vi "Read Power DVR FIFO.vi"(8 "error in (no error)":errorcluster, 9 "Timeout (ms)":i32=100, 10 "Data In":refnum<data-value>[](array[refnum]), 11 "CIFTag in":refnum<class "CIF_NIChn_Fifo_Power_DVR.lvclass">) -> (0 "error out":errorcluster, 1 "timed out?":bool, 2 "Data Out":refnum<data-value>[](array[refnum]), 3 "CIFTag out":refnum<class "CIF_NIChn_Fifo_Power_DVR.lvclass">, 4 "Header":T1)   [LabVIEW 2021, in "CIF_NIChn_Fifo_Power_DVR.lvclass"]
uses:
  CIF_NIChn_Fifo_Power_DVR.lvclass
  CIFChannels/Typedef/Direction.ctl
  CIFChannels/CIFChannels.lvclass
  CIFChannels/Typedef/Channel State.ctl
  NIChn/CIF_NIChn.lvclass
  D:/dev/CIF-LVCore/src/Channels/CIF_NIChn/NIChn/CIF_NIChn.lvclass
  ChannelCommon/typedef/FIFO Header.ctl
  ChannelCommon/ChannelCommon.lvlib
  ChannelCommon/typedef/Datatype Waveform.ctl
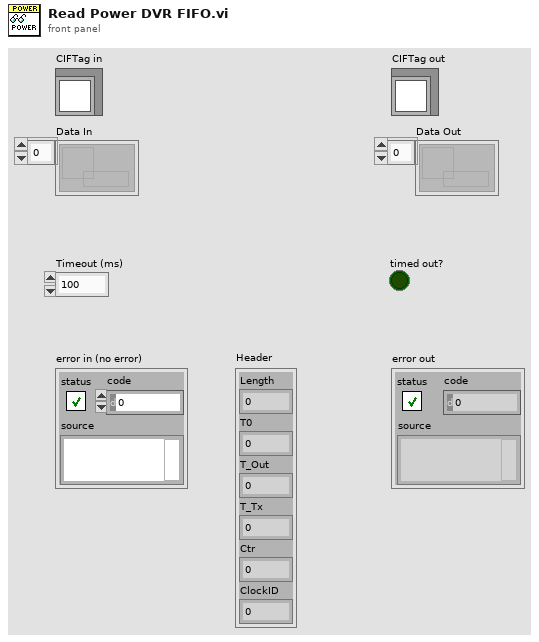
[diagram p1: front panel]
types:
  T1 = typedef "ChannelCommon.lvlib/FIFO Header.ctl" = cluster{"Length":u64, "T0":i64, "T_Out":i64, "T_Tx":i64, "Ctr":u64, "ClockID":u8}
  T2 = typedef "CIFChannels.lvclass/Channel State.ctl" = enum16{"Creating", "Disconnected", "Connecting", "Connected", "Destroyed"}
  T3 = typedef "CIFChannels.lvclass/Direction.ctl" = enum16{"Publisher", "Subscriber"}
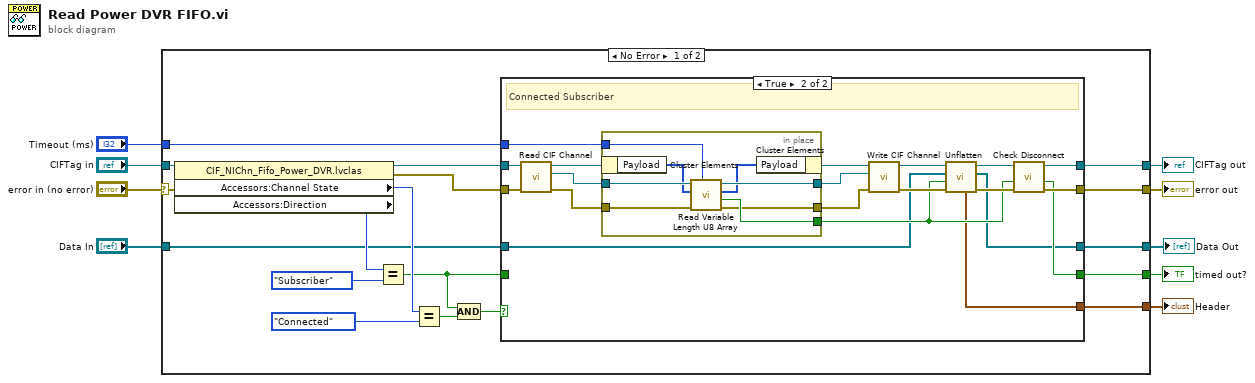
[diagram p0: block diagram]
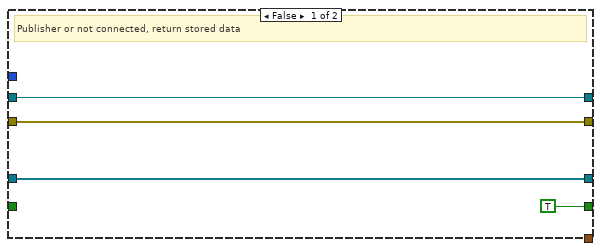
[diagram p2: hidden frame]
diagram:
  n1 = case shown="No Error" "error in (no error)" {
    selector: "error in (no error)" -> [w24 w62]
    tunnel: [w13 w62] -> w8
    tunnel: [w14 w61] -> w6
    tunnel: "CIFTag in" -> [w25 w61]
    tunnel: [w27 _] -> w5
    tunnel: [w26 w60] -> w2
    tunnel: "Timeout (ms)" -> [w12 _]
    tunnel: [w11 _] -> w3
    tunnel: "Data In" -> [w10 w60]
    frame No Error {
      n2 = property class="CIF_NIChn_Fifo_Power_DVR.lvclas"(reference=w25, error in=w24) -> (reference out=w23:refnum<class "CIF_NIChn_Fifo_Power_DVR.lvclass">, error out=w22:errorcluster, "Accessors:Channel State"=w19:T2, "Accessors:Direction"=w21:T3)
      n3 = Equal?(x=w21, y=Direction."Subscriber") -> (x = y?=w15:bool)
      n4 = Equal?(x=w19, y=Channel_State."Connected") -> (x = y?=w17:bool)
      n5 = Compound Arithmetic op=AND(w15, w17) -> (w16:bool)
      n6 = case shown="True" w16 {
        tunnel: [TRUE ("timeout out") w41] -> w27
        tunnel: [w28 w34] -> w26
        tunnel: w22 -> [w30 w50]
        tunnel: w23 -> [w31 w51]
        tunnel: w15 -> [_ _]
        tunnel: [w31 w49] -> w14
        tunnel: [w30 w48] -> w13
        tunnel: w12 -> [_ w40]
        tunnel: [_ w33] -> w11
        tunnel: w10 -> [w28 w32]
        frame False {
          # "Publisher or not connected, return stored data"
        }
        frame True {
          # "Connected Subscriber"
          n7 = call "Read CIF Channel.vi"("error in (no error)"=w50, "CIFTag in"=w51) -> ("error out"=w45:errorcluster, "CIF Channel"=w46:refnum<k21>, "CIFTag out"=w47:refnum<class "CIF_NIChn_Fifo_Power_DVR.lvclass">)  [unwired: 7 in]
          n8 = in-place {
            in-place-border: [w57] -> w35
            in-place-border: w46 -> [w59]
            in-place-border: w45 -> [w58]
            in-place-border: [w56] -> w42
            in-place-border: [w55] -> w43
            in-place-border: w40 -> [w54]
            n9 = in-place-cluster #1(w47) -> ("Payload"=w53:u8[])
            n10 = call <vilib>:"Read Variable Length U8 Array.vi"("Timeout (ms)"=w54, "error in"=w58, "Payload in"=w53, "CIF Channel in"=w59) -> ("error out"=w55:errorcluster, "Timed out?"=w57:bool, "Payload out"=w52:u8[], "CIF Channel out"=w56:refnum<k21>)  [unwired: 4 in]
            n11 = in-place-cluster #1("Payload"=w52) -> (w44:refnum<class "CIF_NIChn_Fifo_Power_DVR.lvclass">)
          }
          n12 = call "Write CIF Channel.vi"("error in (no error)"=w43, "CIF Channel"=w42, "CIFTag in"=w44) -> ("error out"=w38:errorcluster, "CIFTag out"=w39:refnum<class "CIF_NIChn_Fifo_Power_DVR.lvclass">)  [unwired: 7 in]
          n13 = call "Unflatten.vi"("error in (no error)"=w38, "timeout in"=w35, "Data In"=w32, "CIFFifoCAN in"=w39) -> ("error out"=w36:errorcluster, "Data Out"=w34:refnum<data-value>[], "CIFFifoCAN out"=w37:refnum<class "CIF_NIChn_Fifo_Power_DVR.lvclass">, "Header"=w33:T1)  [unwired: 4 in]
          n14 = call "Check Disconnect.vi"("error in (no error)"=w36, "timeout in"=w35, "CIFTag in"=w37) -> ("error out"=w48:errorcluster, "timeout out"=w41:bool, "CIFTag out"=w49:refnum<class "CIF_NIChn_Fifo_Power_DVR.lvclass">)  [unwired: 5 in, 1 out]
        }
      }
    }
    frame Error {
    }
  }
  "error out" <- w8
  "CIFTag out" <- w6
  "timed out?" <- w5
  "Header" <- w3
  "Data Out" <- w2
